vi "read tag name.vi"(8 "error in":errorcluster, 11 "system tag in":refnum<class "data bus tag description.lvclass">) -> (0 "error out":errorcluster, 2 "name":string, 3 "system tag out":refnum<class "data bus tag description.lvclass">)   [LabVIEW 2013, in "data bus tag description.lvclass"]
doc: "Reads the name of the tag, as stored in the tag descriptor."
uses:
  data bus tag description.lvclass
  data bus tag description.lvclass/data bus tag description.ctl
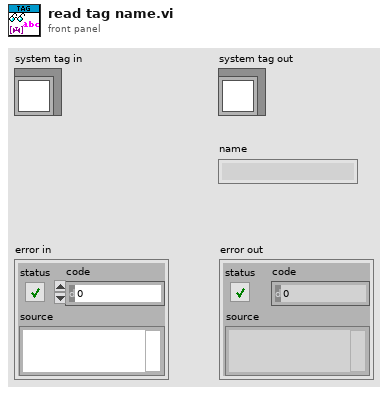
[diagram p1: front panel]
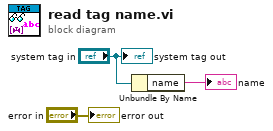
[diagram p0: block diagram]
diagram:
  n1 = Unbundle By Name("system tag in") -> ("name"=→"name":string)
  "system tag out" <- "system tag in"
  "error out" <- "error in"
